vi "TiePie.Lib.init.vi"(8 "error in (no error)":errorcluster) -> (0 "error out":errorcluster)   [LabVIEW 2013, in "LVTiePie.lvlib"]
uses:
  LVTiePie.lvlib
  bin/libtiepie.dll
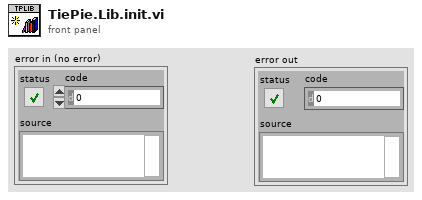
[diagram p1: front panel]
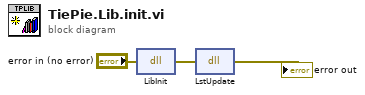
[diagram p0: block diagram]
diagram:
  n1 = dll-call lib="D:/Documents and Settings/XP/Moje dokumenty/acas/trunk/support_projects/ACAS_QY/sources/drivers/LVTiePie/bin/libtiepie.dll" fn="LibInit"(error in="error in (no error)") -> (error out=w2:errorcluster)  [unwired: 3 in, 1 out]
  n2 = dll-call lib="D:/Documents and Settings/XP/Moje dokumenty/acas/trunk/support_projects/ACAS_QY/sources/drivers/LVTiePie/bin/libtiepie.dll" fn="LstUpdate"(error in=w2) -> (error out=→"error out":errorcluster)  [unwired: 3 in, 1 out]
